vi "FRCts20_Backend_Competition_DELETE.vi"(6 "Message Attributes":T4, 8 "error in (no error)":errorcluster, 10 "Data":string, 11 "Engine_Refnums":T1) -> (0 "error out":errorcluster)   [LabVIEW 2013]
doc: "Deletes a competition. This also deletes any divisions associated with it, as divisions are children of competitions. Called by the competition/division api, and expects a competition name."
uses:
  Dependencies/Keyed Array/KeyedArray.ctl
  FRCts20_Backend_EngineRefnums.ctl
  INI_Accessor/FRCts20_Backend_INI Controller.lvclass
  Dependencies/AMC/_SubVIs/TypeDefs/Message Queue.ctl
  Dependencies/AMC/_SubVIs/TypeDefs/Message.ctl
  <vilib>/addons/database/Connection.llb/Conn ObjectReference.ctl
  FRCts20_Backend_FGVOperation.ctl
  FRCts20_Backend_API/FRCts20_Backend_API_Competition.ctl
  FRCts20_Backend_Engine.lvlib
  FRCts20_Backend_API/FRCts20_Backend_API.lvlib
  Dependencies/Keyed Array/Tools_KeyedArray.lvlib
  Dependencies/AMC/AMC.lvlib
  <vilib>/addons/database/NI_Database_API.lvlib
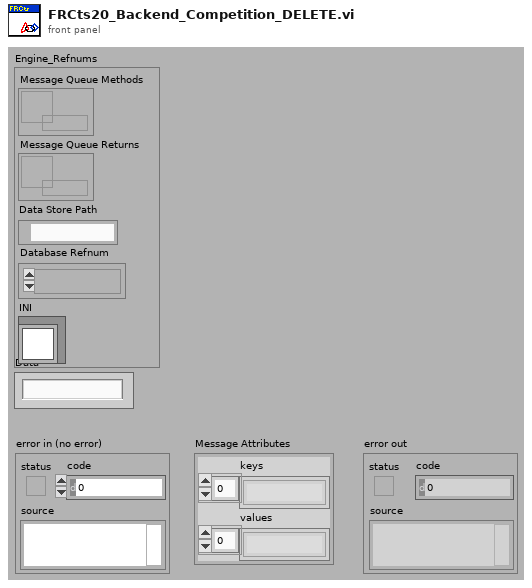
[diagram p1: front panel]
types:
  T1 = typedef "FRCts20_Backend_Engine.lvlib/FRCts20_Backend_EngineRefnums.ctl" = cluster{"Message Queue Methods":T2, "Message Queue Returns":T2, "Data Store Path":path, "Database Refnum":T3, "INI":refnum<class "FRCts20_Backend_INI Controller.lvclass">}
  T2 = typedef "AMC.lvlib/Message Queue.ctl" = refnum<queue>
  T3 = typedef "NI_Database_API.lvlib/Conn ObjectReference.ctl" = refnum<k1>
  T4 = typedef "Tools_KeyedArray.lvlib/KeyedArray.ctl" = cluster{"keys":string[], "values":string[]}
  T5 = typedef "FRCts20_Backend_API.lvlib/FRCts20_Backend_API_Competition.ctl" = cluster{"Name":string, "Start Date":timestamp, "Duration":u8, "Divisions":string[], "APIReturn":string}
  T6 = typedef "FRCts20_Backend_Engine.lvlib/FRCts20_Backend_FGVOperation.ctl" = enum16{"Initialize", "EnqueueMessage", "EnqueueDataReturn", "FlushMessage", "FlushDataReturn"}
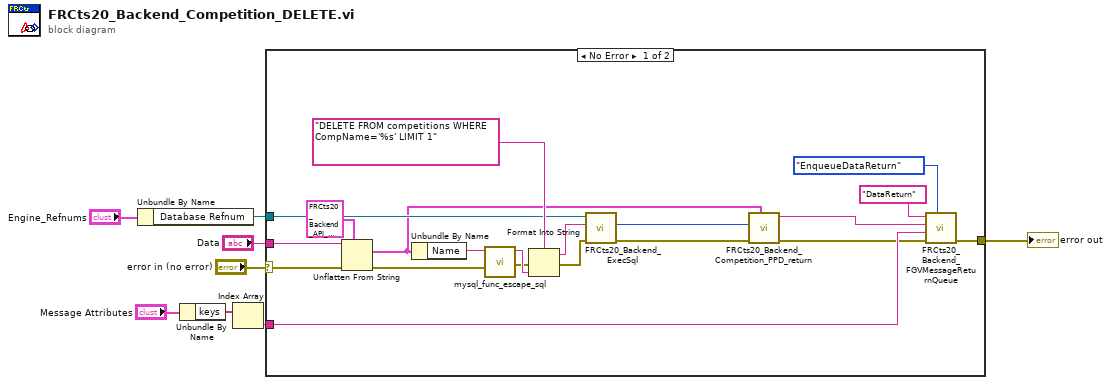
[diagram p0: block diagram]
diagram:
  n1 = Unbundle By Name("Engine_Refnums") -> ("Database Refnum"=w5:T3)
  n2 = Unbundle By Name("Message Attributes") -> ("keys"=w2:string[])
  n3 = Index Array(array=w2) -> (element=w1:string)  [unwired: 1 in]
  n4 = case shown="No Error" "error in (no error)" {
    selector: "error in (no error)" -> [w25 w29]
    tunnel: [w28 w29] -> w7
    tunnel: w5 -> [w15 _]
    tunnel: "Data" -> [w26 _]
    tunnel: w1 -> [w27 _]
    frame No Error {
      n5 = Unflatten From String(type=T5 {"Name"="", "Start Date"=timestamp(0 s since 1904-01-01), "Duration"=0, "Divisions"=[], "APIReturn"=""} ("Competition"), binary string=w26, error in (no error)=w25) -> (value=w10:T5, error out=w17:errorcluster)  [unwired: 2 in, 1 out]
      n6 = Unbundle By Name(w10) -> ("Name"=w19:string)
      n7 = call "mysql_func_escape_sql.vi"("error in (no error)"=w17, "sqlin"=w19) -> ("error out"=w16:errorcluster, "escaped"=w18:string)  [unwired: 8 in]
      n8 = Format Into String(format string="DELETE FROM competitions WHERE CompName='%s' LIMIT 1", error in=w16, w18) -> (resulting string=w14:string, error out=w13:errorcluster)  [unwired: 1 in]
      n9 = call "FRCts20_Backend_ExecSql.vi"("error in (no error)"=w13, "format string"=w14, "Refnum in"=w15) -> ("error out"=w12:errorcluster, "rows affected"=w9:i32)  [unwired: 6 in, 1 out]
      n10 = call "FRCts20_Backend_Competition_PPD_return.vi"("Competition"=w10, "error in (no error)"=w12, "rows affected"=w9) -> ("error out"=w20:errorcluster, "data string"=w21:string)  [unwired: 7 in]
      n11 = call "FRCts20_Backend_FGVMessageReturnQueue.vi"("Operation"=FRCts20_Backend_FGVOperation."EnqueueDataReturn", "error in (no error)"=w20, "Key"=w27, "Message Value"=w21, "Message Name"="DataReturn") -> ("error out"=w28:errorcluster)  [unwired: 5 in, 1 out]
    }
    frame Error {
    }
  }
  "error out" <- w7
